vi "系统设置_古田户外.vi"() -> ()   [LabVIEW 2016]
uses:
  <vilib>/Utility/miscctls.llb/LVPointTypeDef.ctl
  <vilib>/Utility/config.llb/NI_LVConfig.lvlib
  <vilib>/ptbypt/NI_PtbyPt.lvlib
panel:
  out "最近一次启动时间":timestamp
  in  "质控启动日期":string(combo)="关闭"
  in  "跨度核查时间":u16(ring)=6 items=["00H", "01H", "02H", "03H", "04H", "05H", "06H", "07H", "08H", "09H", "10H", "11H", "12H", "13H", "14H", "15H", "16H", "17H", "18H", "19H", "20H", "21H", "22H", "23H"]
  in  "空白核查时间":u16(ring)=2 items=["00H", "01H", "02H", "03H", "04H", "05H", "06H", "07H", "08H", "09H", "10H", "11H", "12H", "13H", "14H", "15H", "16H", "17H", "18H", "19H", "20H", "21H", "22H", "23H"]
  in  "运行模式":enum16{"维护模式", "常规模式", "应急模式", "质控模式"}(ring)
  in  "运行间隔":i16=4 min=1 max=24
  # "质控频次："
  # "空白核查时间："
  # "跨度核查时间："
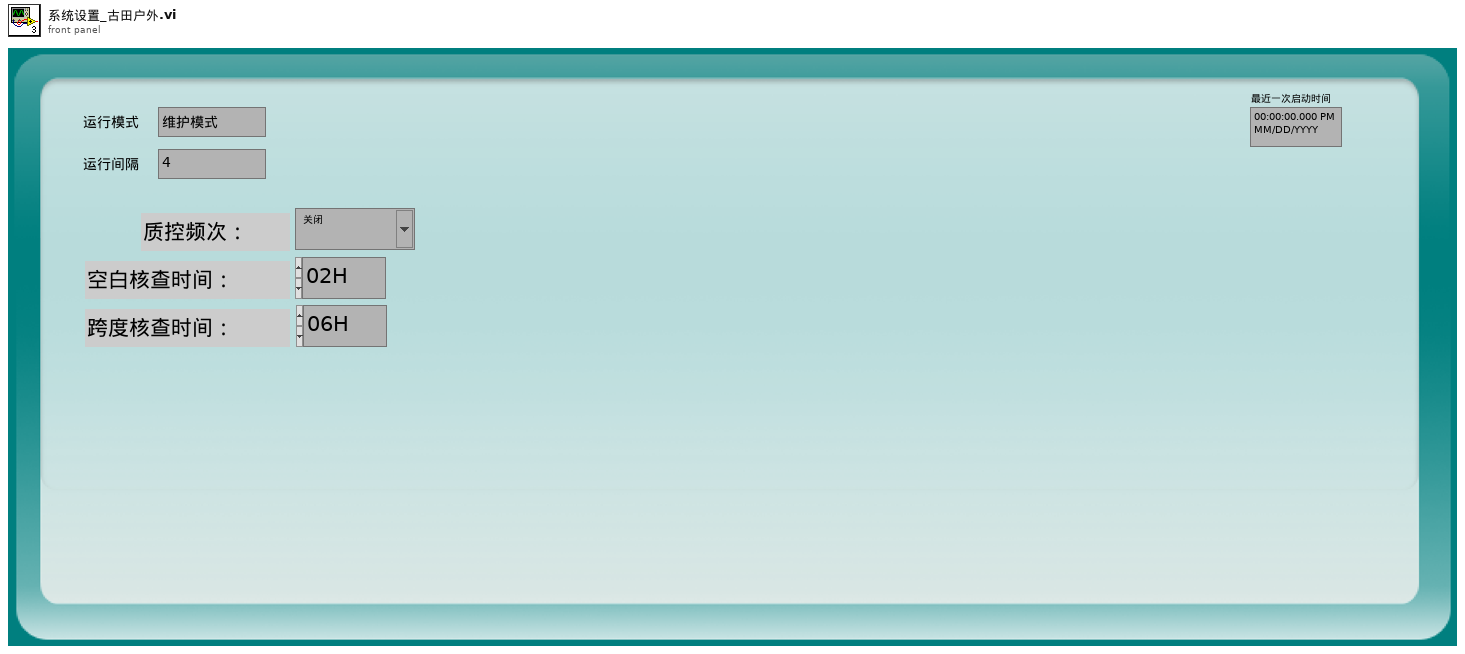
[diagram p1: front panel]
types:
  T1 = typedef "LVPointTypeDef.ctl" = cluster{"Horizontal":i16, "Vertical":i16}
  T2 = typedef "NI_LVConfig.lvlib/Config Data RefNum.ctl" = refnum<k1>
  T3 = cluster{"测量模式":enum16{"水样测量", "标样核查", "零点核查", "跨度核查", "空白测试", "加标回收", "平行样", "校零", "校标"}}
  T4 = cluster{"水样测试量程切换模式":enum16{"H", "L", "AUTO"}, "空白核查量程切换模式":enum16{"H", "L", "AUTO"}, "跨度核查量程切换模式":enum16{"H", "L", "AUTO"}}
  T5 = cluster{"站号":u16, "量程切换":enum32{"H", "L", "AUTO"}, "控制命令":enum16{"启动测量", "标样核查", "零点核查", "跨度核查", "空白测试", "平行样测试", "加标回收", "空白校准", "标样校准", "初始化（清洗）", "停止测试", "仪器重启", "校时", "模式设置", "测量间隔设置"}, "模式设置":enum16{"待机", "连续模式", "周期模式", "定点模式", "受控模式", "手动模式"}, "测量间隔":u16}
  T6 = enum16{"水样测量", "标样核查", "零点核查", "跨度核查", "空白测试", "加标回收", "平行样", "校零", "校标"}
  T7 = cluster{"是否启用仪器":bool, "启动测量模式":cluster{"测量模式":enum16{"水样测量", "标样核查", "零点核查", "跨度核查", "空白测试", "加标回收", "平行样", "校零", "校标"}}, "CODMn":cluster{"确定按钮":bool}}
  T8 = typedef "LVDateTimeRec.ctl" = cluster{"秒数的小数部分":dbl, "秒":i32, "分":i32, "时":i32, "日":i32, "月":i32, "年":i32, "天数（周）":i32, "天数（年）":i32, "DST":i32}
  T9 = enum32{"Bad", "Idle", "Run top level", "Running"}
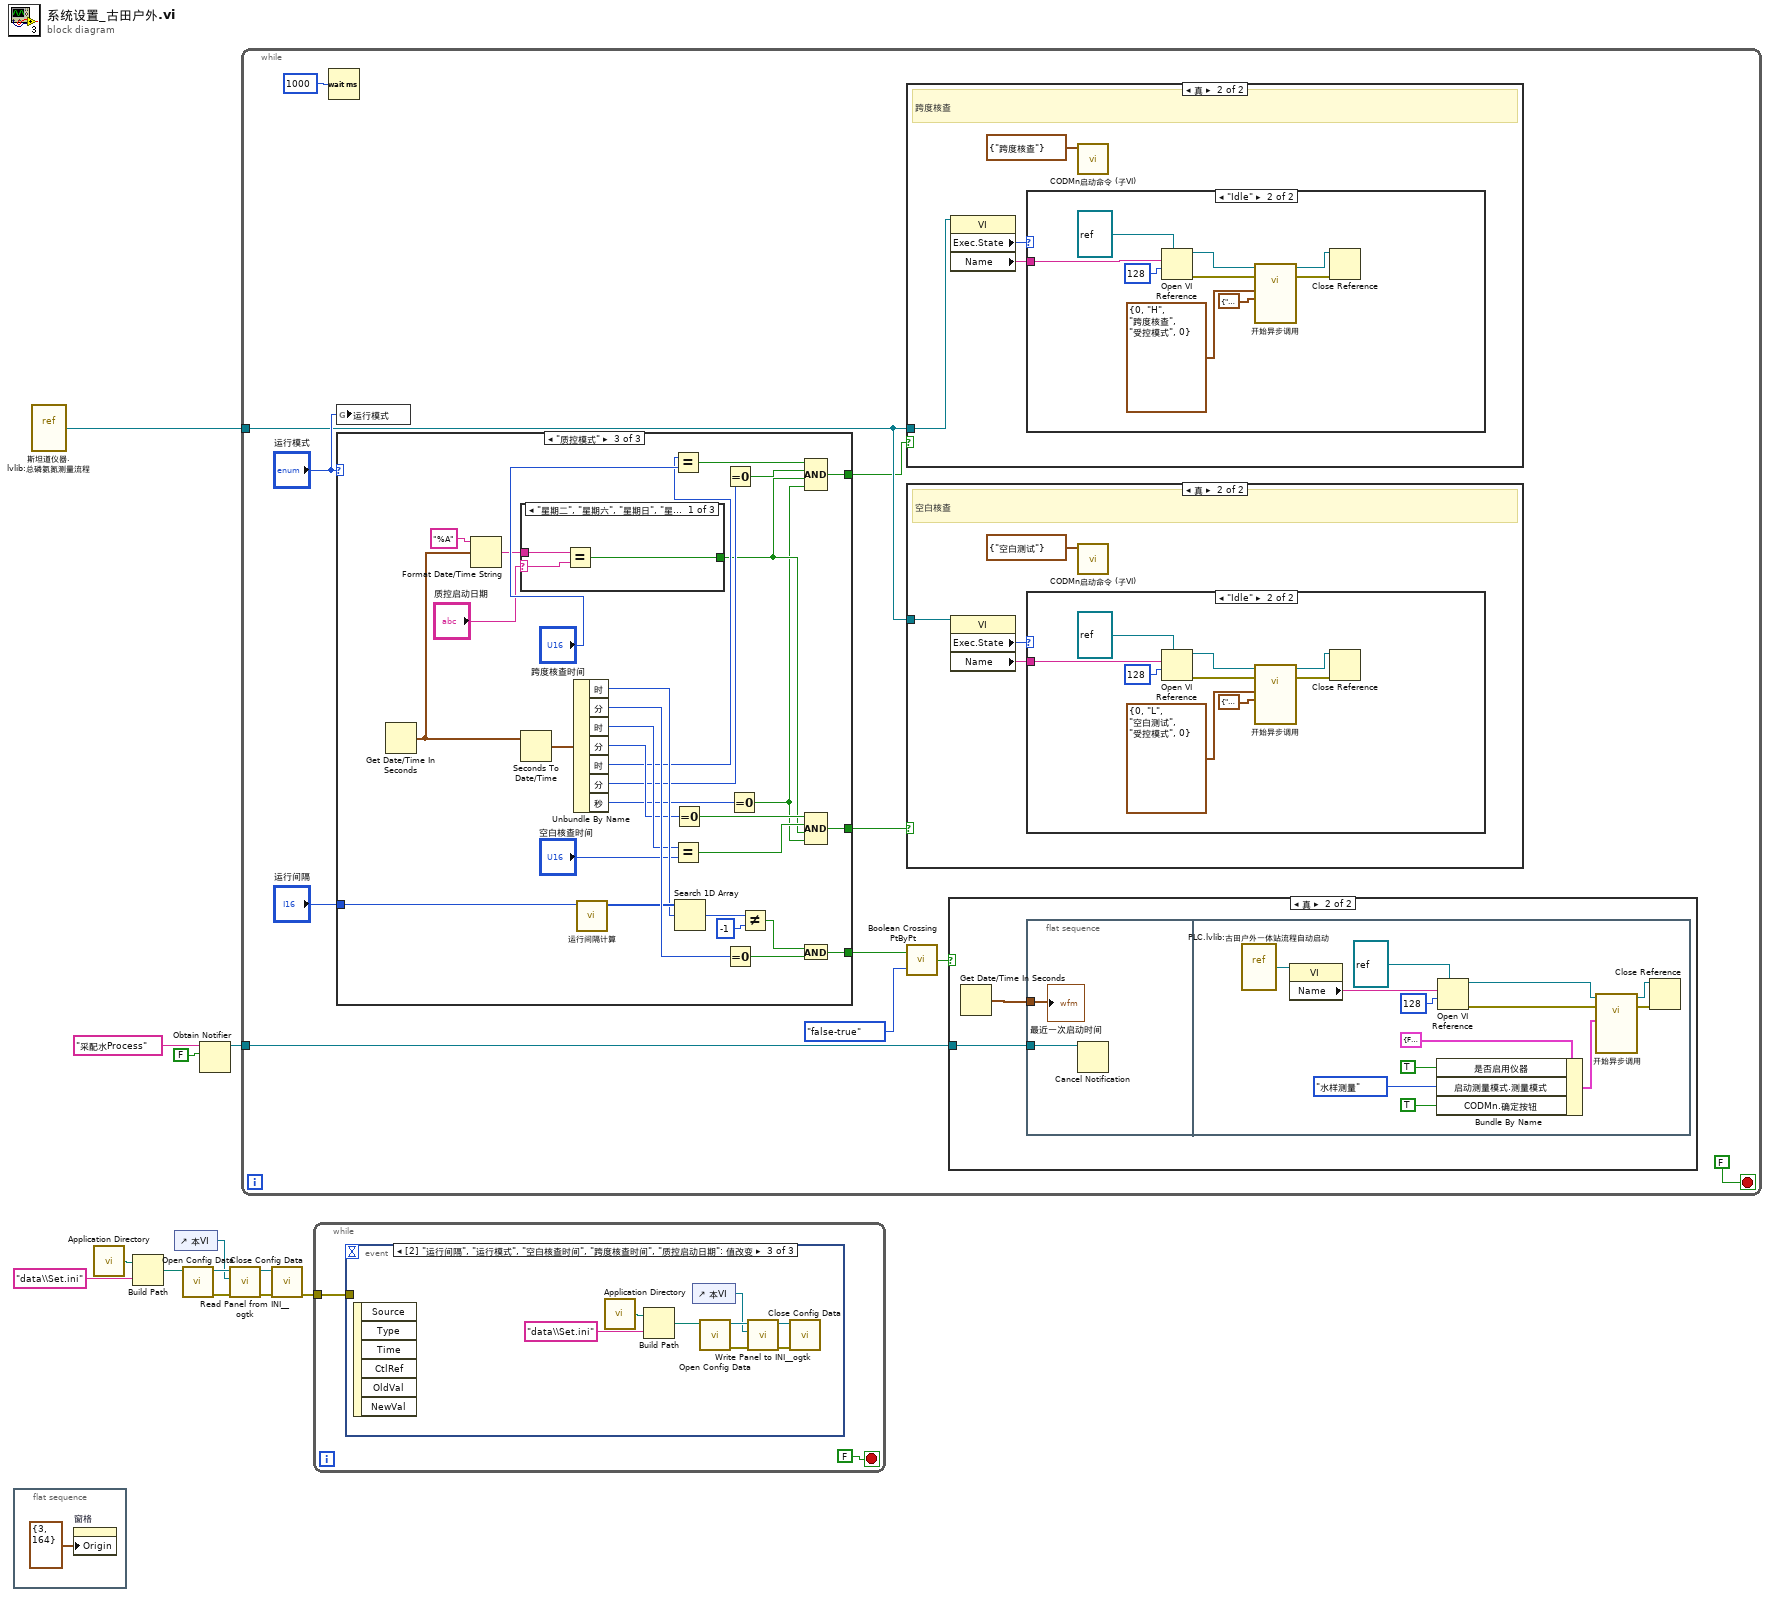
[diagram p0: block diagram]
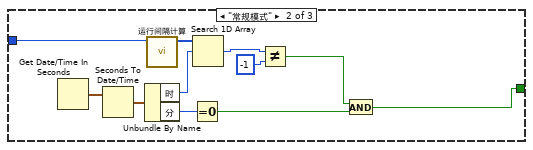
[diagram p8: hidden frame]
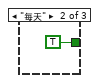
[diagram p9: hidden frame]
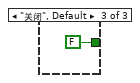
[diagram p10: hidden frame]
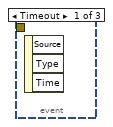
[diagram p11: hidden frame]
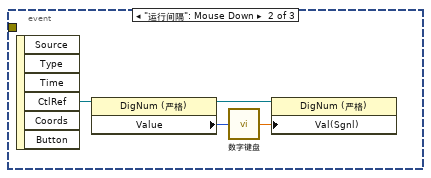
[diagram p12: hidden frame]
diagram:
  n1 = flat-sequence {
    frame #0 {
      n2 = property on="窗格" class="Pane"("Origin"=T1 {"Horizontal"=3, "Vertical"=164} ("原点")) -> ()  [unwired: 2 in, 2 out]
    }
  }
  n3 = vi-ref "斯坦道仪器.lvlib:总磷氨氮测量流程.vi"() -> (w1:refnum<vi>)
  n4 = call <vilib>:"Application Directory.vi"() -> ("Application Directory"=w10:path)
  n5 = Build Path(base path=w10, name or relative path="data\\Set.ini" ("名称或相对路径")) -> (appended path=w8:path)
  n6 = control-ref of="本VI"() -> (w2:refnum<vi>)
  n7 = call <vilib>:"Open Config Data.vi"("configuration file path"=w8) -> ("error out"=w5:errorcluster, "refnum"=w6:T2)  [unwired: 8 in, 1 out]
  n8 = Obtain Notifier(name (unnamed)="采配水Process" ("名称（未命名）"), notification data type=FALSE) -> (notifier out=w11:refnum<notifier>)  [unwired: 2 in, 2 out]
  n9 = call <userlib>:"Read Panel from INI__ogtk.vi"("error in (no error)"=w5, "VI ref"=w2, "refnum"=w6) -> ("error out"=w4:errorcluster, "refnum out"=w3:T2)  [unwired: 7 in]
  n10 = while {
    tunnel: w11 -> [w23]
    tunnel: w1 -> [w19]
    stop <- FALSE stop-if-true
    n11 = Wait (ms)(milliseconds to wait=u32 1000 ("等待时间（毫秒）")) -> ()  [unwired: 1 out]
    n12 = global write "系统变量.vi" "运行模式"("运行模式") -> ()
    n13 = case shown="\"质控模式\"" "运行模式" {
      tunnel: [_ w70 w100] -> w17
      tunnel: "运行间隔" -> [_ w69 w99]
      tunnel: [_ _ w93] -> w20
      tunnel: [_ _ w87] -> w18
      frame "维护模式", Default {
      }
      frame "常规模式" {
        n14 = Get Date/Time In Seconds() -> (seconds since 1Jan1904=w79:timestamp)
        n15 = Seconds To Date/Time(time stamp (now)=w79) -> (date time rec=w78:T8)  [unwired: 1 in]
        n16 = Unbundle By Name(w78) -> ("时"=w75:i32, "分"=w77:i32)
        n17 = call "运行间隔计算.vi"("运行周期"=w69) -> ("数组"=w76:i32[])  [unwired: 10 in]
        n18 = Equal To 0?(x=w77) -> (x = 0?=w71:bool)
        n19 = Search 1D Array(1D array=w76, element=w75) -> (index of element=w74:i32)  [unwired: 1 in]
        n20 = Not Equal?(x=w74, y=-1) -> (x != y?=w72:bool)
        n21 = And(x=w72, y=w71) -> (x .and. y?=w70:bool)
      }
      frame "质控模式" {
        n22 = Get Date/Time In Seconds() -> (seconds since 1Jan1904=w84:timestamp)
        n23 = Format Date/Time String(time format string (%c)="%A" ("时间格式字符串(%c)"), seconds (now)=w84) -> (date/time string=w82:string)  [unwired: 1 in]
        n24 = case shown="\"星期二\", \"星期六\", \"星期日\", \"星期三\", \"星期四\", \"星期五\", \"星期一\"" "质控启动日期" {
          selector: "质控启动日期" -> [w111 _ _]
          tunnel: [w110 TRUE FALSE] -> w85
          tunnel: w82 -> [w109 _ _]
          frame "星期二", "星期六", "星期日", "星期三", "星期四", "星期五", "星期一" {
            n25 = Equal?(x=w109, y=w111) -> (x = y?=w110:bool)
          }
          frame "每天" {
          }
          frame "关闭", Default {
          }
        }
        n26 = Seconds To Date/Time(time stamp (now)=w84) -> (date time rec=w108:T8)  [unwired: 1 in]
        n27 = Unbundle By Name(w108) -> ("时"=w105:i32, "分"=w107:i32, "时"=w98:i32, "分"=w96:i32, "时"=w91:i32, "分"=w90:i32, "秒"=w81:i32)
        n28 = call "运行间隔计算.vi"("运行周期"=w99) -> ("数组"=w106:i32[])  [unwired: 10 in]
        n29 = Equal?(x=w91, y="跨度核查时间") -> (x = y?=w89:bool)
        n30 = Equal?(x=w98, y="空白核查时间") -> (x = y?=w95:bool)
        n31 = Equal To 0?(x=w96) -> (x = 0?=w94:bool)
        n32 = Search 1D Array(1D array=w106, element=w105) -> (index of element=w104:i32)  [unwired: 1 in]
        n33 = Equal To 0?(x=w90) -> (x = 0?=w88:bool)
        n34 = Equal To 0?(x=w107) -> (x = 0?=w101:bool)
        n35 = Equal To 0?(x=w81) -> (x = 0?=w80:bool)
        n36 = Not Equal?(x=w104, y=-1) -> (x != y?=w102:bool)
        n37 = And(x=w102, y=w101) -> (x .and. y?=w100:bool)
        n38 = Compound Arithmetic op=AND ("复合运算")(w89, w88, w85, w80) -> (w87:bool)
        n39 = Compound Arithmetic op=AND ("复合运算")(w94, w95, w85, w80) -> (w93:bool)
      }
    }
    n40 = case shown="真" w18 {
      tunnel: w19 -> [_ w29]
      frame False {
      }
      frame True {
        # "跨度核查"
        n41 = property class="VI"(reference=w29) -> ("Exec.State"=w28:T9, "Name"=w27:string)  [unwired: 1 in, 2 out]
        n42 = case shown="\"Idle\"" w28 {
          tunnel: w27 -> [_ w38]
          frame "Bad", Default {
          }
          frame "Idle" {
            n43 = Open VI Reference(type specifier VI Refnum (for type only)=refnum<vi> refnum ("类型说明符VI引用句柄（仅用于类型）"), vi path=w38, options=128 ("选项")) -> (vi reference=w35:refnum<vi>, error out=w31:errorcluster)  [unwired: 3 in]
            n44 = call-by-ref "开始异步调用"(reference=w35, error in=w31, "量程模式"=T4 {"水样测试量程切换模式"=enum."AUTO", "空白核查量程切换模式"=enum."AUTO", "跨度核查量程切换模式"=enum."AUTO"}, "参数"=T5 {"站号"=0, "量程切换"=enum."H", "控制命令"=enum."跨度核查", "模式设置"=enum."受控模式", "测量间隔"=0}) -> (reference out=w32:refnum<vi>, error out=w30:errorcluster)  [unwired: 10 in]
            n45 = Close Reference(reference=w32, error in (no error)=w30) -> ()  [unwired: 1 out]
          }
        }
        n46 = call "CODMn启动命令 (子VI).vi"("启动测量模式"=T3 {"测量模式"=enum."跨度核查"}) -> ()  [unwired: 11 in]
      }
    }
    n47 = case shown="真" w20 {
      tunnel: w19 -> [_ w42]
      frame False {
      }
      frame True {
        # "空白核查"
        n48 = property class="VI"(reference=w42) -> ("Exec.State"=w41:T9, "Name"=w40:string)  [unwired: 1 in, 2 out]
        n49 = case shown="\"Idle\"" w41 {
          tunnel: w40 -> [_ w51]
          frame "Bad", Default {
          }
          frame "Idle" {
            n50 = Open VI Reference(type specifier VI Refnum (for type only)=refnum<vi> refnum ("类型说明符VI引用句柄（仅用于类型）"), vi path=w51, options=128 ("选项")) -> (vi reference=w48:refnum<vi>, error out=w44:errorcluster)  [unwired: 3 in]
            n51 = call-by-ref "开始异步调用"(reference=w48, error in=w44, "量程模式"=T4 {"水样测试量程切换模式"=enum."AUTO", "空白核查量程切换模式"=enum."AUTO", "跨度核查量程切换模式"=enum."AUTO"}, "参数"=T5 {"站号"=0, "量程切换"=enum."L", "控制命令"=enum."空白测试", "模式设置"=enum."受控模式", "测量间隔"=0}) -> (reference out=w45:refnum<vi>, error out=w43:errorcluster)  [unwired: 10 in]
            n52 = Close Reference(reference=w45, error in (no error)=w43) -> ()  [unwired: 1 out]
          }
        }
        n53 = call "CODMn启动命令 (子VI).vi"("启动测量模式"=T3 {"测量模式"=enum."空白测试"}) -> ()  [unwired: 11 in]
      }
    }
    n54 = call <vilib>:"Boolean Crossing PtByPt.vi"("direction"=enum16{"either", "false-true", "true-false"}."false-true", "input"=w17) -> ("crossing"=w16:bool)  [unwired: 1 in]
    n55 = case shown="真" w16 {
      tunnel: w23 -> [_ w53]
      frame False {
      }
      frame True {
        n56 = Get Date/Time In Seconds() -> (seconds since 1Jan1904=w52:timestamp)
        n57 = flat-sequence {
          tunnel: w53 -> [w55]
          tunnel: w52 -> [w54]
          frame #0 {
            n58 = Cancel Notification(0:w55) -> ()  [unwired: 1 in, 3 out]
            "最近一次启动时间" <- w54
          }
          frame #1 {
            n59 = vi-ref "PLC.lvlib:古田户外一体站流程自动启动.vi"() -> (w68:refnum<vi>)
            n60 = property class="VI"(reference=w68) -> ("Name"=w67:string)  [unwired: 1 in, 2 out]
            n61 = Bundle By Name(cluster=T7 {"是否启用仪器"=FALSE, "启动测量模式"={"测量模式"=enum."水样测量"}, "CODMn"={"确定按钮"=FALSE}} ("参数"), "是否启用仪器"=TRUE, "启动测量模式.测量模式"=T6."水样测量", "CODMn.确定按钮"=TRUE) -> (w56:T7)
            n62 = Open VI Reference(type specifier VI Refnum (for type only)=refnum<vi> refnum, vi path=w67, options=128 ("选项")) -> (vi reference=w65:refnum<vi>, error out=w62:errorcluster)  [unwired: 3 in]
            n63 = call-by-ref "开始异步调用"(reference=w65, error in=w62, "参数"=w56) -> (reference out=w63:refnum<vi>, error out=w61:errorcluster)  [unwired: 11 in]
            n64 = Close Reference(reference=w63, error in (no error)=w61) -> ()  [unwired: 1 out]
          }
        }
      }
    }
  }
  n65 = call <vilib>:"Close Config Data.vi"("error in (no error)"=w4, "refnum"=w3) -> ("error out"=w7:errorcluster)  [unwired: 8 in, 1 out]
  n66 = while {
    tunnel: w7 -> [w114]
    stop <- FALSE stop-if-true
    n67 = event shown="[2] \"运行间隔\", \"运行模式\", \"空白核查时间\", \"跨度核查时间\", \"质控启动日期\": 值改变" {
      selector: _ -> [_ _ _]
      dyn-events: _ -> [_ _ _]
      timeout: _ -> [_ _ _]
      tunnel: w114 -> [_ _ _]
      event Timeout {
        n68 = event-data() -> ()  [unwired: 1 in, 3 out]
      }
      event "运行间隔": Mouse Down {
        n69 = event-data() -> ("CtlRef"=w116:refnum<vi>)  [unwired: 1 in, 5 out]
        n70 = property class="DigNum (严格)"(reference=w116) -> (reference out=w118:refnum<vi>, "Value"=w117:i16)  [unwired: 1 in, 1 out]
        n71 = call "数字键盘.vi"("OldNumber"=w117) -> ("NewNumber"=w119:sgl)
        n72 = property class="DigNum (严格)"(reference=w118, "Val(Sgnl)"=w119) -> ()  [unwired: 1 in, 2 out]
      }
      event "运行间隔", "运行模式", "空白核查时间", "跨度核查时间", "质控启动日期": Value Change {
        n73 = event-data() -> ()  [unwired: 1 in, 6 out]
        n74 = call <vilib>:"Application Directory.vi"() -> ("Application Directory"=w127:path)
        n75 = Build Path(base path=w127, name or relative path="data\\Set.ini" ("名称或相对路径")) -> (appended path=w125:path)
        n76 = control-ref of="本VI"() -> (w120:refnum<vi>)
        n77 = call <vilib>:"Open Config Data.vi"("configuration file path"=w125) -> ("error out"=w123:errorcluster, "refnum"=w124:T2)  [unwired: 8 in, 1 out]
        n78 = call <userlib>:"Write Panel to INI__ogtk.vi"("error in (no error)"=w123, "VI ref"=w120, "refnum"=w124) -> ("error out"=w121:errorcluster, "refnum out"=w122:T2)  [unwired: 7 in]
        n79 = call <vilib>:"Close Config Data.vi"("error in (no error)"=w121, "refnum"=w122) -> ()  [unwired: 8 in, 2 out]
      }
    }
  }
